vi "Update.vi"(8 "error in (no error)":errorcluster, 11 "Example Source in":refnum<class "Example Source.lvclass">) -> (0 "error out":errorcluster, 3 "Example Source out":refnum<class "Example Source.lvclass">)   [LabVIEW 2016, in "Example Source.lvlib" / "Example Source.lvclass"]
uses:
  Example Source.lvclass
  C:/Projects/Shared Libraries/Event Actors/Event Source/Event Source.lvclass
  C:/Program Files (x86)/National Instruments/LabVIEW 2016/vi.lib/ActorFramework/Actor/Actor.lvclass
  Example Events/Double Array Event.lvclass
  C:/Projects/Shared Libraries/Event Actors/Event/Event.lvclass
  Example Events/Timestamp Event.lvclass
  Event/Event.lvclass/Event.ctl
  <vilib>/ActorFramework/Actor/Actor.lvclass/Actor.ctl
  <vilib>/ActorFramework/Message Enqueuer/Message Enqueuer.lvclass/Message Enqueuer.ctl
  Example Events/Timestamp Event.lvclass/Timestamp Event.ctl
  Example Events/Double Array Event.lvclass/Double Array Event.ctl
  Event Source Messages/Generate Event Msg/Generate Event Msg.lvclass/Generate Event Msg.ctl
  <vilib>/ActorFramework/Message Enqueuer/Init from Existing Queue.vi
  <vilib>/ActorFramework/Message Enqueuer/Enqueue.vi
  Event Source Messages/Generate Event Msg/Generate Event Msg.lvclass
  C:/Program Files (x86)/National Instruments/LabVIEW 2016/vi.lib/ActorFramework/Message/Message.lvclass
  <vilib>/Utility/LVClass/Get LV Class Name.vi
  <resource>/AFDebug/Generate Trace for Message.vi
  <vilib>/ActorFramework/Message Priority Queue/Priority Enqueue.vi
  <vilib>/ActorFramework/Message Enqueuer/Message Enqueuer.lvclass
  <vilib>/ActorFramework/Actor/Actor.lvclass
  Event Source/Event Source.lvclass
  Event/Event.lvclass
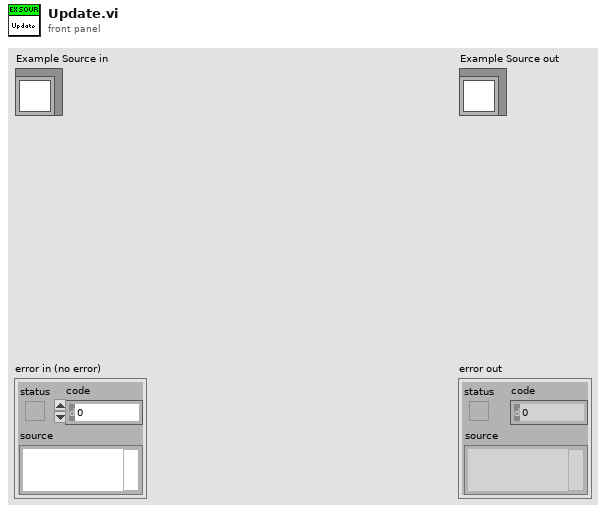
[diagram p1: front panel]
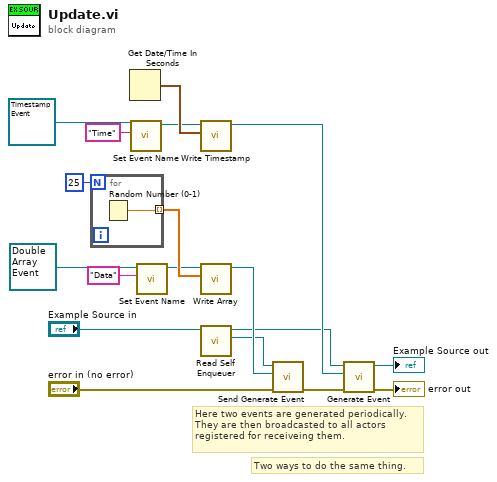
[diagram p0: block diagram]
diagram:
  # "Two ways to do the same thing."
  # "Here two events are generated periodically.\nThey are then broadcasted to all actors \nregistered for receiveing them."
  n1 = for {
    N: 25 -> [_]
    tunnel: [w18] -> w15 mode=indexing
    n2 = Random Number (0-1)() -> (number: 0 to 1=w18:dbl)
  }
  n3 = Get Date/Time In Seconds() -> (seconds since 1Jan1904=w17:timestamp)
  n4 = call "Set Event Name.vi"("Name (Generic)"="Time", "Event In"=refnum<class "Timestamp Event.lvclass"> refnum ("Timestamp Event out")) -> ("Event Out"=w5:refnum<class "Timestamp Event.lvclass">)  [unwired: 9 in]
  n5 = call "Set Event Name.vi"("Name (Generic)"="Data", "Event In"=refnum<class "Double Array Event.lvclass"> refnum ("Double Array Event out")) -> ("Event Out"=w9:refnum<class "Double Array Event.lvclass">)  [unwired: 9 in]
  n6 = call "Write Timestamp.vi"("Timestamp"=w17, "Timestamp Event in"=w5) -> ("Timestamp Event out"=w10:refnum<class "Timestamp Event.lvclass">)  [unwired: 9 in]
  n7 = call "Write Array.vi"("Array"=w15, "Double Array Event in"=w9) -> ("Double Array Event out"=w13:refnum<class "Double Array Event.lvclass">)  [unwired: 9 in]
  n8 = call <vilib>:"Read Self Enqueuer.vi"("Actor"="Example Source in") -> ("Self Enqueuer"=w12:refnum<class "Message Enqueuer.lvclass">)  [unwired: 10 in]
  n9 = call "Send Generate Event.vi"("error in (no error)"="error in (no error)", "Event"=w13, "Message Enqueuer in"=w12) -> ("error out"=w11:errorcluster)  [unwired: 7 in, 1 out]
  n10 = call "Generate Event.vi"("Error In"=w11, "Event"=w10, "Event Source In"="Example Source in") -> ("Error Out"=→"error out":errorcluster, "Event Source Out"=→"Example Source out":refnum<class "Example Source.lvclass">)  [unwired: 7 in]
